vi "ROI entry-Init palette type.vi"(8 "error in (no error)":errorcluster) -> (0 "error out":errorcluster)   [LabVIEW 2020]
uses:
  ROI Entry screen/Globals/gl_ROI Entry UI globals.vi
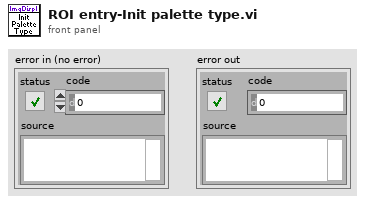
[diagram p1: front panel]
types:
  T1 = typedef "ROI entry screen ctrl refs cluster.ctl" = cluster{"Done button":refnum<vi>, "Imaging button":refnum<vi>, "Acquisition button":refnum<vi>, "Scan dwell time per pixel (us)":refnum<vi>, "# of planes":refnum<vi>, "Zoom Ctrl":refnum<vi>, "Equal size":refnum<vi>, "Channel":refnum<vi>, "Image Display":refnum<vi>, "Z-Plane Selector":refnum<vi>, "Number of lines left":refnum<vi>, "Z-stack folder path":refnum<vi>, "POI Density":refnum<vi>, "Arb Plane Entry":refnum<vi>, "Whole Plane":refnum<vi>, "Line Mode":refnum<vi>, "Clear Last":refnum<vi>, "Clear All":refnum<vi>, "Delete Lines":refnum<vi>, "Trial Length (sec)":refnum<vi>, "Palette Type":refnum<vi>, "Intensity slider":refnum<vi>, "# POI":refnum<vi>, "Max Z Proj":refnum<vi>, "Zplane ind":refnum<vi>, "Wavelength (nm)":refnum<vi>, "Number of Trials":refnum<vi>, "Funct stim.trig.enable":refnum<vi>, "Funct stim.trig.delay (s)":refnum<vi>, "Line Mode":refnum<vi>, "Step size (µm)":refnum<vi>, "ROI move mode":refnum<vi>, "Cool-down time (s)":refnum<vi>, "Enable cool-down time":refnum<vi>, "Motor Z ind. (um)":refnum<vi>, "AOL Z ind. (um)":refnum<vi>, "Load Reference Image":refnum<vi>, "Rel.  Res.":refnum<vi>, "ROI LIST":refnum<vi>, "Show All":refnum<vi>, "ROI Type":refnum<vi>, "Start Plane":refnum<vi>, "Stop Plane":refnum<vi>, "Offset ROI":refnum<vi>, "Tab Control":refnum<vi>, "Laser Power(%)":refnum<vi>, "Cycle rate":refnum<vi>, "FOV (Ind.)":refnum<vi>, "Frame Size (Ind.)":refnum<vi>, "Resolution (Ind.)":refnum<vi>, "Pixel Density (Ind)":refnum<vi>, "Laser Power (Ind.)":refnum<vi>, "Dwell Time (Ind.)":refnum<vi>, "Adj MC":refnum<vi>}
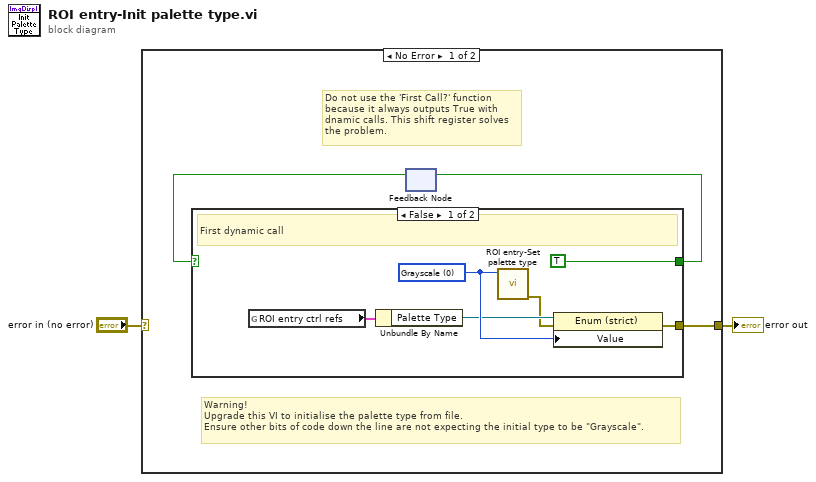
[diagram p0: block diagram]
diagram:
  n1 = case shown="No Error" "error in (no error)" {
    selector: "error in (no error)" -> [_ w13]
    tunnel: [w3 w13] -> w2
    frame No Error {
      # "Warning!\nUpgrade this VI to initialise the palette type from file.\nEnsure other bits of code down the line are not expecting the initial type to be \"Grayscale\"."
      # "Do not use the 'First Call?' function because it always outputs True with dnamic calls. This shift register solves the problem."
      n2 = feedback #1() -> (w4:bool)  [unwired: 1 in]
      n3 = case shown="False" w4 {
        selector: w4 -> [_ w12]
        tunnel: [TRUE w12] -> w5
        tunnel: [w6 _] -> w3
        frame False {
          w10 = u32 0 items=["Grayscale", "Binary", "Gradient", "Rainbow", "Temperature", "User Defined"] ("Palette:Palette Type")
          # "First dynamic call"
          n4 = global read "gl_ROI Entry UI globals.vi" "ROI entry ctrl refs"() -> (w9:T1)
          n5 = Unbundle By Name(w9) -> ("Palette Type"=w8:refnum<vi>)
          n6 = call "ROI entry-Set palette type.vi"("Palette:Palette Type"=w10) -> ("error out"=w7:errorcluster)  [unwired: 10 in]
          n7 = property class="Enum (strict)"(reference=w8, error in=w7, "Value"=w10) -> (error out=w6:errorcluster)  [unwired: 1 out]
        }
        frame True {
        }
      }
      n8 = feedback-in #1(w5) -> ()
    }
    frame Error {
    }
  }
  "error out" <- w2
